vi "Round_off_current_values.vi"(6 "Numeric 4":dbl, 9 "Numeric 3":dbl, 10 "Numeric 2":dbl, 11 "Numeric":dbl) -> (1 "Current 3":dbl, 2 "Current 2":dbl, 3 "Current 1":dbl, 4 "Current 4":dbl)   [LabVIEW 2011]
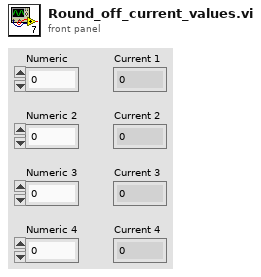
[diagram p1: front panel]
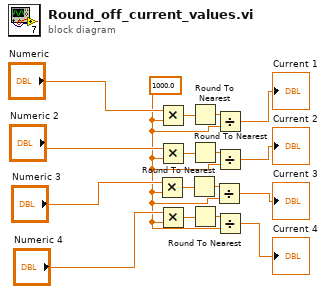
[diagram p0: block diagram]
diagram:
  w9 = 1000.0 ("y")
  n1 = Multiply(x="Numeric 3", y=w9) -> (x*y=w5:dbl)
  n2 = Multiply(x="Numeric", y=w9) -> (x*y=w1:dbl)
  n3 = Multiply(x="Numeric 2", y=w9) -> (x*y=w4:dbl)
  n4 = Multiply(x="Numeric 4", y=w9) -> (x*y=w7:dbl)
  n5 = Round To Nearest(number=w5) -> (nearest integer value=w6:dbl)
  n6 = Round To Nearest(number=w1) -> (nearest integer value=w2:dbl)
  n7 = Round To Nearest(number=w4) -> (nearest integer value=w3:dbl)
  n8 = Round To Nearest(number=w7) -> (nearest integer value=w8:dbl)
  n9 = Divide(x=w6, y=w9) -> (x/y=→"Current 3":dbl)
  n10 = Divide(x=w2, y=w9) -> (x/y=→"Current 1":dbl)
  n11 = Divide(x=w3, y=w9) -> (x/y=→"Current 2":dbl)
  n12 = Divide(x=w8, y=w9) -> (x/y=→"Current 4":dbl)
